vi "Format Seconds to Uptime String.vi"(11 "Elapsed Time (s)":dbl) -> (3 "Uptime String":string)   [LabVIEW 2019]
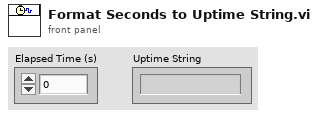
[diagram p1: front panel]
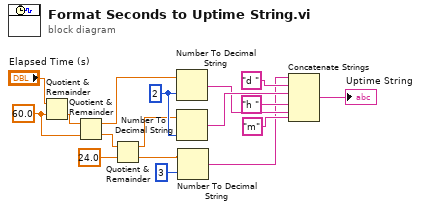
[diagram p0: block diagram]
diagram:
  w16 = i16 2 ("width (-)")
  w3 = 60.0 ("y")
  n1 = Quotient & Remainder(x="Elapsed Time (s)", y=w3) -> (floor(x/y)=w1:dbl)  [unwired: 1 out]
  n2 = Quotient & Remainder(x=w1, y=w3) -> (x-y*floor(x/y)=w10:dbl, floor(x/y)=w2:dbl)
  n3 = Quotient & Remainder(x=w2, y=24.0) -> (x-y*floor(x/y)=w8:dbl, floor(x/y)=w15:dbl)
  n4 = Number To Decimal String(number=w10, width (-)=w16) -> (decimal integer string=w9:string)
  n5 = Number To Decimal String(number=w8, width (-)=w16) -> (decimal integer string=w17:string)
  n6 = Number To Decimal String(number=w15, width (-)=i16 3) -> (decimal integer string=w5:string)
  n7 = Concatenate Strings(w5, "d " ("string"), w17, "h " ("string"), w9, "m" ("string")) -> (→"Uptime String":string)
